vi "Request StatusFGV.vi"(8 "Error In":errorcluster, 11 "Command":enum16{"Block", "Unblock", "Check Status"}(ring)) -> (0 "Error Out":errorcluster, 3 "Blocked?":bool)   [LabVIEW 2017, in "Client.lvlib" / "CommsServer.lvlib"]
uses:
  CommsServer.lvlib
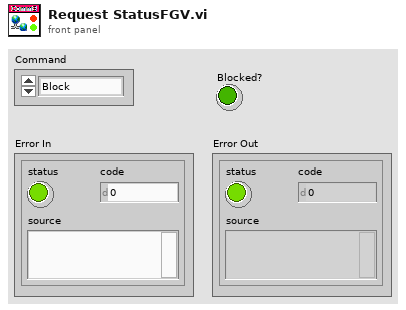
[diagram p1: front panel]
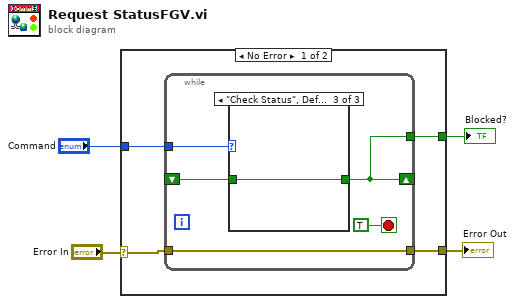
[diagram p0: block diagram]
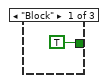
[diagram p2: hidden frame]
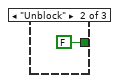
[diagram p3: hidden frame]
diagram:
  n1 = case shown="No Error" "Error In" {
    selector: "Error In" -> [w6 w17]
    tunnel: "Command" -> [w8 _]
    tunnel: [w5 w17] -> w2
    tunnel: [w7 _] -> w1
    frame No Error {
      n2 = while {
        tunnel: w8 -> [w12]
        shift-right: [w10] -> _
        shift-left: _ -> [w11]
        tunnel: [w10] -> w7
        tunnel: w6 -> [w9]
        tunnel: [w9] -> w5
        stop <- TRUE stop-if-true
        n3 = case shown="\"Check Status\", Default" w12 {
          tunnel: [TRUE FALSE w16] -> w10
          tunnel: w11 -> [_ _ w16]
          frame "Block" {
          }
          frame "Unblock" {
          }
          frame "Check Status", Default {
          }
        }
      }
    }
    frame Error {
    }
  }
  "Error Out" <- w2
  "Blocked?" <- w1
